vi "Standard_Error_Est.vi"(2 "N":dbl, 3 "4th order moment u^4":dbl, 4 "2nd order moment u^2":dbl) -> (0 "Standard error in variance":dbl, 1 "Standard error in Mean":dbl)   [LabVIEW 2020]
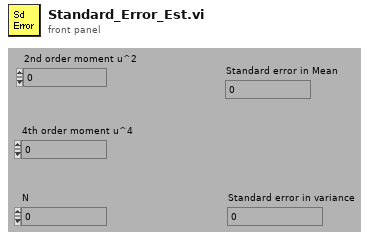
[diagram p1: front panel]
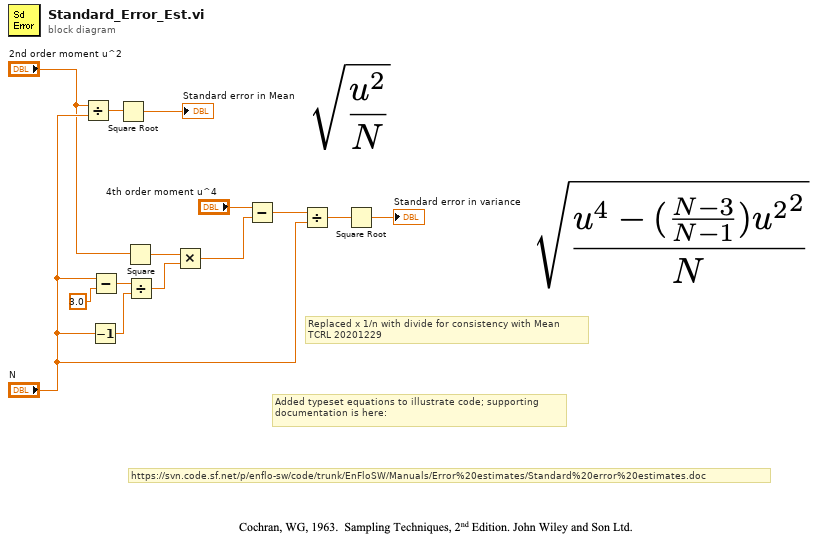
[diagram p0: block diagram]
diagram:
  # "https://svn.code.sf.net/p/enflo-sw/code/trunk/EnFloSW/Manuals/Error%20estimates/Standard%20error%20estimates.doc"
  # "Replaced x 1/n with divide for consistency with Mean\nTCRL 20201229"
  # "Added typeset equations to illustrate code; supporting documentation is here:"
  n1 = Divide(x="2nd order moment u^2", y="N") -> (x/y=w14:dbl)
  n2 = Decrement(x="N") -> (x-1=w10:dbl)
  n3 = Subtract(x="N", y=3.0) -> (x-y=w11:dbl)
  n4 = Square Root(x=w14) -> (sqrt(x)=→"Standard error in Mean":dbl)
  n5 = Square(x="2nd order moment u^2") -> (x^2=w7:dbl)
  n6 = Divide(x=w11, y=w10) -> (x/y=w9:dbl)
  n7 = Multiply(x=w7, y=w9) -> (x*y=w6:dbl)
  n8 = Subtract(x="4th order moment u^4", y=w6) -> (x-y=w4:dbl)
  n9 = Divide(x=w4, y="N") -> (x/y=w3:dbl)
  n10 = Square Root(x=w3) -> (sqrt(x)=→"Standard error in variance":dbl)
